vi "2019 deep space game Final.vi"() -> ()   [LabVIEW 2018]
panel:
  in  "Red Auto Points":dbl
  in  "Red End Game Points":dbl
  out "Red Score":dbl(slide) scale=0.0..200.0
  in  "Red Hatch":bool
  in  "Red Cargo":bool
  in  "Blue Foul":bool
  in  "Blue Tech Foul":bool
  out "Blue Score":dbl(slide) scale=0.0..200.0
  in  "Red Tech Foul":bool
  in  "Red Foul":bool
  in  "Blue End Game Points":dbl
  in  "Blue Auto Points":dbl
  in  "Blue Cargo":bool
  in  "Blue Hatch":bool
  out "Red Table of Pain":dbl[](array[numeric])
  out "Blue Table of Pain":dbl[](array[numeric])
  out "Thunder Down Under":T1
  out "SHARP":T1
  out "MARS":T1
  out "CIA":T1
  out "Cheezy Poofs":T1
  in  "End Game":bool
  out "Turn Number":i32(slide) scale=0.0..30.0
  in  "Next Turn":bool
  out "Krios":T1
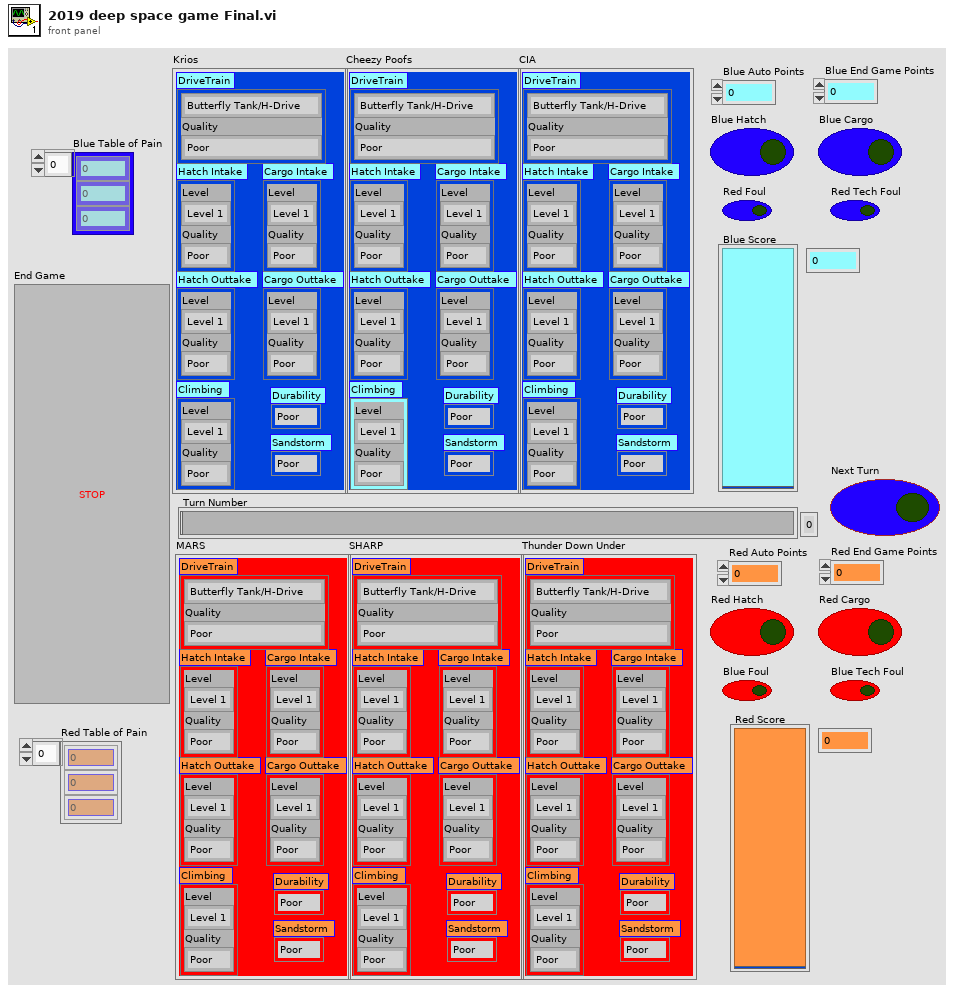
[diagram p1: front panel]
types:
  T1 = cluster{"DriveTrain":cluster{enum16{"Butterfly Tank/H-Drive", "Butterfly-Tank/Tank", "Tread", "Strafe", "Swerve", "Tank Traction"}, "Quality":enum16{"Poor", "Good", "Excellent"}}, "Cargo Intake":cluster{"Level":enum16{"Level 1", "Level 2", "Level 3"}, "Quality":enum16{"Poor", "Good", "Excellent"}}, "Hatch Intake":cluster{"Level":enum16{"Level 1", "Level 2", "Level 3"}, "Quality":enum16{"Poor", "Good", "Excellent"}}, "Cargo Outtake":cluster{"Level":enum16{"Level 1", "Level 2", "Level 3"}, "Quality":enum16{"Poor", "Good", "Excellent"}}, "Hatch Outtake":cluster{"Level":enum16{"Level 1", "Level 2", "Level 3"}, "Quality":enum16{"Poor", "Good", "Excellent"}}, "Climbing":cluster{"Level":enum16{"Level 1", "Level 2", "Level 3"}, "Quality":enum16{"Poor", "Good", "Excellent"}}, "Durability":enum16{"Poor", "Good", "Excellent"}, "Sandstorm":enum16{"Poor", "Good", "Excellent"}}
  T2 = cluster{cluster{enum16{"Butterfly Tank/H-Drive", "Butterfly-Tank/Tank", "Tread", "Strafe", "Swerve", "Tank Traction"}, "y":enum16{"Poor", "Good", "Excellent"}}, cluster{"Level":enum16{"Level 1", "Level 2", "Level 3"}, "y":enum16{"Poor", "Good", "Excellent"}}, cluster{"Level":enum16{"Level 1", "Level 2", "Level 3"}, "y":enum16{"Poor", "Good", "Excellent"}}, cluster{"Level":enum16{"Level 1", "Level 2", "Level 3"}, "y":enum16{"Poor", "Good", "Excellent"}}, cluster{"Level":enum16{"Level 1", "Level 2", "Level 3"}, "y":enum16{"Poor", "Good", "Excellent"}}, "Climbing":cluster{"Level":enum16{"Level 1", "Level 2", "Level 3"}, "Quality":enum16{"Poor", "Good", "Excellent"}}, "Durability":enum16{"Poor", "Good", "Excellent"}, "Sandstorm":enum16{"Poor", "Good", "Excellent"}}
  T3 = cluster{"Sandstorm":cluster{cluster{enum16{"Butterfly Tank/H-Drive", "Butterfly-Tank/Tank", "Tread", "Strafe", "Swerve", "Tank Traction"}, "y":enum16{"Poor", "Good", "Excellent"}}, cluster{"Level":enum16{"Level 1", "Level 2", "Level 3"}, "y":enum16{"Poor", "Good", "Excellent"}}, cluster{"Level":enum16{"Level 1", "Level 2", "Level 3"}, "y":enum16{"Poor", "Good", "Excellent"}}, cluster{"Level":enum16{"Level 1", "Level 2", "Level 3"}, "y":enum16{"Poor", "Good", "Excellent"}}, cluster{"Level":enum16{"Level 1", "Level 2", "Level 3"}, "y":enum16{"Poor", "Good", "Excellent"}}, "Climbing":cluster{"Level":enum16{"Level 1", "Level 2", "Level 3"}, "Quality":enum16{"Poor", "Good", "Excellent"}}, "Durability":enum16{"Poor", "Good", "Excellent"}, "Sandstorm":enum16{"Poor", "Good", "Excellent"}}, "Sandstorm":cluster{cluster{enum16{"Butterfly Tank/H-Drive", "Butterfly-Tank/Tank", "Tread", "Strafe", "Swerve", "Tank Traction"}, "y":enum16{"Poor", "Good", "Excellent"}}, cluster{"Level":enum16{"Level 1", "Level 2", "Level 3"}, "y":enum16{"Poor", "Good", "Excellent"}}, cluster{"Level":enum16{"Level 1", "Level 2", "Level 3"}, "y":enum16{"Poor", "Good", "Excellent"}}, cluster{"Level":enum16{"Level 1", "Level 2", "Level 3"}, "y":enum16{"Poor", "Good", "Excellent"}}, cluster{"Level":enum16{"Level 1", "Level 2", "Level 3"}, "y":enum16{"Poor", "Good", "Excellent"}}, "Climbing":cluster{"Level":enum16{"Level 1", "Level 2", "Level 3"}, "Quality":enum16{"Poor", "Good", "Excellent"}}, "Durability":enum16{"Poor", "Good", "Excellent"}, "Sandstorm":enum16{"Poor", "Good", "Excellent"}}, "Sandstorm":cluster{cluster{enum16{"Butterfly Tank/H-Drive", "Butterfly-Tank/Tank", "Tread", "Strafe", "Swerve", "Tank Traction"}, "y":enum16{"Poor", "Good", "Excellent"}}, cluster{"Level":enum16{"Level 1", "Level 2", "Level 3"}, "y":enum16{"Poor", "Good", "Excellent"}}, cluster{"Level":enum16{"Level 1", "Level 2", "Level 3"}, "y":enum16{"Poor", "Good", "Excellent"}}, cluster{"Level":enum16{"Level 1", "Level 2", "Level 3"}, "y":enum16{"Poor", "Good", "Excellent"}}, cluster{"Level":enum16{"Level 1", "Level 2", "Level 3"}, "y":enum16{"Poor", "Good", "Excellent"}}, "Climbing":cluster{"Level":enum16{"Level 1", "Level 2", "Level 3"}, "Quality":enum16{"Poor", "Good", "Excellent"}}, "Durability":enum16{"Poor", "Good", "Excellent"}, "Sandstorm":enum16{"Poor", "Good", "Excellent"}}, "Sandstorm":cluster{cluster{enum16{"Butterfly Tank/H-Drive", "Butterfly-Tank/Tank", "Tread", "Strafe", "Swerve", "Tank Traction"}, "y":enum16{"Poor", "Good", "Excellent"}}, cluster{"Level":enum16{"Level 1", "Level 2", "Level 3"}, "y":enum16{"Poor", "Good", "Excellent"}}, cluster{"Level":enum16{"Level 1", "Level 2", "Level 3"}, "y":enum16{"Poor", "Good", "Excellent"}}, cluster{"Level":enum16{"Level 1", "Level 2", "Level 3"}, "y":enum16{"Poor", "Good", "Excellent"}}, cluster{"Level":enum16{"Level 1", "Level 2", "Level 3"}, "y":enum16{"Poor", "Good", "Excellent"}}, "Climbing":cluster{"Level":enum16{"Level 1", "Level 2", "Level 3"}, "Quality":enum16{"Poor", "Good", "Excellent"}}, "Durability":enum16{"Poor", "Good", "Excellent"}, "Sandstorm":enum16{"Poor", "Good", "Excellent"}}, "Sandstorm":cluster{cluster{enum16{"Butterfly Tank/H-Drive", "Butterfly-Tank/Tank", "Tread", "Strafe", "Swerve", "Tank Traction"}, "y":enum16{"Poor", "Good", "Excellent"}}, cluster{"Level":enum16{"Level 1", "Level 2", "Level 3"}, "y":enum16{"Poor", "Good", "Excellent"}}, cluster{"Level":enum16{"Level 1", "Level 2", "Level 3"}, "y":enum16{"Poor", "Good", "Excellent"}}, cluster{"Level":enum16{"Level 1", "Level 2", "Level 3"}, "y":enum16{"Poor", "Good", "Excellent"}}, cluster{"Level":enum16{"Level 1", "Level 2", "Level 3"}, "y":enum16{"Poor", "Good", "Excellent"}}, "Climbing":cluster{"Level":enum16{"Level 1", "Level 2", "Level 3"}, "Quality":enum16{"Poor", "Good", "Excellent"}}, "Durability":enum16{"Poor", "Good", "Excellent"}, "Sandstorm":enum16{"Poor", "Good", "Excellent"}}, "Sandstorm":cluster{cluster{enum16{"Butterfly Tank/H-Drive", "Butterfly-Tank/Tank", "Tread", "Strafe", "Swerve", "Tank Traction"}, "y":enum16{"Poor", "Good", "Excellent"}}, cluster{"Level":enum16{"Level 1", "Level 2", "Level 3"}, "y":enum16{"Poor", "Good", "Excellent"}}, cluster{"Level":enum16{"Level 1", "Level 2", "Level 3"}, "y":enum16{"Poor", "Good", "Excellent"}}, cluster{"Level":enum16{"Level 1", "Level 2", "Level 3"}, "y":enum16{"Poor", "Good", "Excellent"}}, cluster{"Level":enum16{"Level 1", "Level 2", "Level 3"}, "y":enum16{"Poor", "Good", "Excellent"}}, "Climbing":cluster{"Level":enum16{"Level 1", "Level 2", "Level 3"}, "Quality":enum16{"Poor", "Good", "Excellent"}}, "Durability":enum16{"Poor", "Good", "Excellent"}, "Sandstorm":enum16{"Poor", "Good", "Excellent"}}}
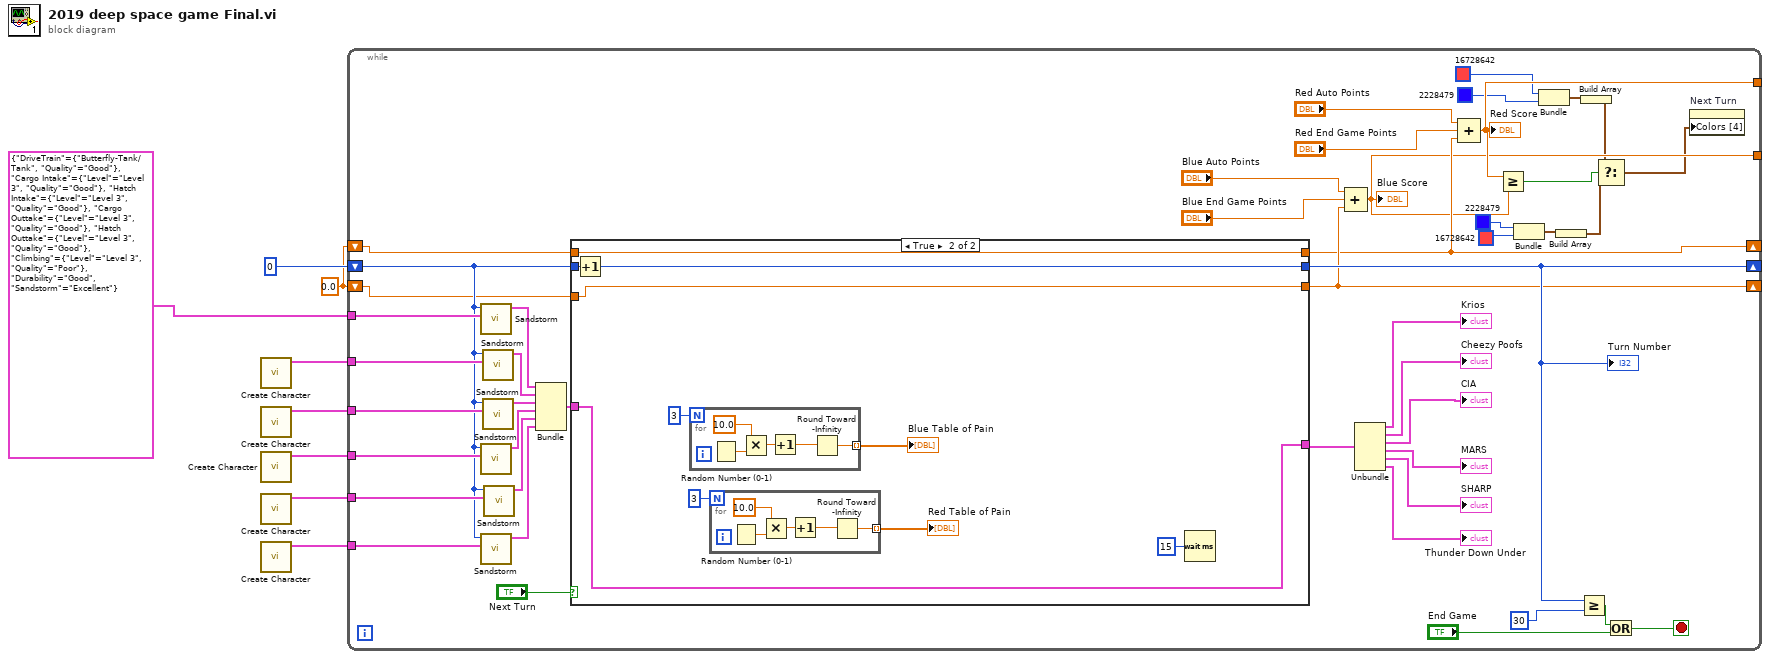
[diagram p0: block diagram]
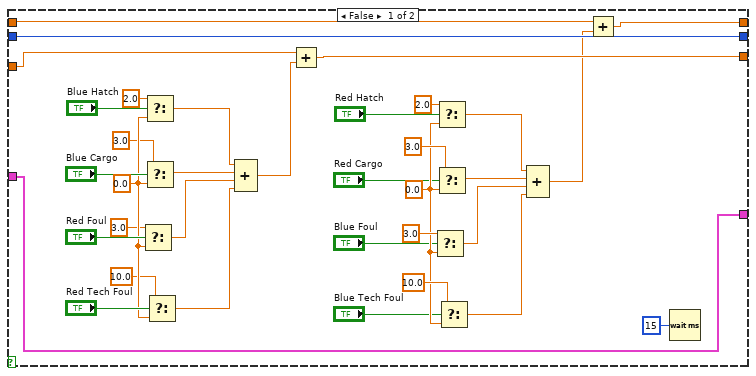
[diagram p2: hidden frame]
diagram:
  w2 = 0.0
  n1 = call "Create Character.vi"() -> ("Normal Game"=w7:T1)  [unwired: 11 in]
  n2 = call "Create Character.vi"() -> ("Normal Game"=w6:T1)  [unwired: 11 in]
  n3 = call "Create Character.vi"() -> ("Normal Game"=w5:T1)  [unwired: 11 in]
  n4 = call "Create Character.vi"() -> ("Normal Game"=w4:T1)  [unwired: 11 in]
  n5 = call "Create Character.vi"() -> ("Normal Game"=w3:T1)  [unwired: 11 in]
  n6 = while {
    shift-right: [w50] -> _
    shift-left: 0 -> [w43]
    tunnel: T1 {"DriveTrain"={enum."Butterfly-Tank/Tank", "Quality"=enum."Good"}, "Cargo Intake"={"Level"=enum."Level 3", "Quality"=enum."Good"}, "Hatch Intake"={"Level"=enum."Level 3", "Quality"=enum."Good"}, "Cargo Outtake"={"Level"=enum."Level 3", "Quality"=enum."Good"}, "Hatch Outtake"={"Level"=enum."Level 3", "Quality"=enum."Good"}, "Climbing"={"Level"=enum."Level 3", "Quality"=enum."Poor"}, "Durability"=enum."Good", "Sandstorm"=enum."Excellent"} ("Normal Game") -> [w44]
    tunnel: w7 -> [w45]
    tunnel: w6 -> [w46]
    tunnel: w5 -> [w47]
    tunnel: w4 -> [w48]
    tunnel: w3 -> [w49]
    shift-right: [w21] -> _
    shift-left: w2 -> [w28]
    shift-right: [w26] -> _
    shift-left: w2 -> [w27]
    tunnel: [w19] -> _
    tunnel: [w18] -> _
    stop <- w54 stop-if-true
    n7 = call "Sandstorm.vi"("Normal Game"=w44, "Turn Number in"=w43) -> ("Sandstorm"=w42:T2)  [unwired: 9 in]
    n8 = call "Sandstorm.vi"("Normal Game"=w47, "Turn Number in"=w43) -> ("Sandstorm"=w37:T2)  [unwired: 9 in]
    n9 = call "Sandstorm.vi"("Normal Game"=w49, "Turn Number in"=w43) -> ("Sandstorm"=w39:T2)  [unwired: 9 in]
    n10 = call "Sandstorm.vi"("Normal Game"=w45, "Turn Number in"=w43) -> ("Sandstorm"=w41:T2)  [unwired: 9 in]
    n11 = call "Sandstorm.vi"("Normal Game"=w46, "Turn Number in"=w43) -> ("Sandstorm"=w40:T2)  [unwired: 9 in]
    n12 = call "Sandstorm.vi"("Normal Game"=w48, "Turn Number in"=w43) -> ("Sandstorm"=w38:T2)  [unwired: 9 in]
    n13 = Bundle("Sandstorm"=w42, "Sandstorm"=w41, "Sandstorm"=w40, "Sandstorm"=w37, "Sandstorm"=w38, "Sandstorm"=w39) -> (w36:T3)  [unwired: 1 in]
    n14 = case shown="True" "Next Turn" {
      tunnel: w43 -> [w90 w100]
      tunnel: [w90 w99] -> w50
      tunnel: w36 -> [w88 w97]
      tunnel: [w88 w97] -> w35
      tunnel: w28 -> [w57 w92]
      tunnel: w27 -> [w74 w91]
      tunnel: [w56 w92] -> w21
      tunnel: [w72 w91] -> w26
      frame False {
        w62 = 0.0 ("f")
        w83 = 0.0 ("f")
        n15 = Select(t=3.0, s="Red Foul", f=w83) -> (s? t:f=w76:dbl)
        n16 = Select(t=2.0, s="Blue Hatch", f=w83) -> (s? t:f=w78:dbl)
        n17 = Select(t=3.0, s="Blue Cargo", f=w83) -> (s? t:f=w77:dbl)
        n18 = Select(t=10.0, s="Red Tech Foul", f=w83) -> (s? t:f=w75:dbl)
        n19 = Compound Arithmetic op=ADD(w78, w77, w76, w75) -> (w73:dbl)
        n20 = Add(x=w74, y=w73) -> (x+y=w72:dbl)
        n21 = Select(t=3.0, s="Blue Foul", f=w62) -> (s? t:f=w69:dbl)
        n22 = Select(t=2.0, s="Red Hatch", f=w62) -> (s? t:f=w67:dbl)
        n23 = Select(t=3.0, s="Red Cargo", f=w62) -> (s? t:f=w68:dbl)
        n24 = Select(t=10.0, s="Blue Tech Foul", f=w62) -> (s? t:f=w70:dbl)
        n25 = Compound Arithmetic op=ADD(w67, w68, w69, w70) -> (w71:dbl)
        n26 = Add(x=w57, y=w71) -> (x+y=w56:dbl)
        n27 = Wait (ms)(milliseconds to wait=u32 15) -> ()  [unwired: 1 out]
      }
      frame True {
        n28 = Increment(x=w100) -> (x+1=w99:i32)
        n29 = for {
          N: 3 -> [_]
          tunnel: [w108] -> w95 mode=indexing
          n30 = Random Number (0-1)() -> (number: 0 to 1=w110:dbl)
          n31 = Multiply(x=10.0, y=w110) -> (x*y=w107:dbl)
          n32 = Increment(x=w107) -> (x+1=w106:dbl)
          n33 = Round Toward -Infinity(1:w106) -> (0:w108:dbl)
        }
        "Blue Table of Pain" <- w95
        n34 = for {
          N: 3 -> [_]
          tunnel: [w103] -> w94 mode=indexing
          n35 = Random Number (0-1)() -> (number: 0 to 1=w105:dbl)
          n36 = Multiply(x=10.0, y=w105) -> (x*y=w102:dbl)
          n37 = Increment(x=w102) -> (x+1=w101:dbl)
          n38 = Round Toward -Infinity(1:w101) -> (0:w103:dbl)
        }
        "Red Table of Pain" <- w94
        n39 = Wait (ms)(milliseconds to wait=u32 15) -> ()  [unwired: 1 out]
      }
    }
    "Turn Number" <- w50
    n40 = Compound Arithmetic op=ADD("Blue Auto Points", "Blue End Game Points", w26) -> (w18:dbl)
    "Blue Score" <- w18
    n41 = Unbundle(w35) -> ("Sandstorm"=→"Krios":T2, "Sandstorm"=→"Cheezy Poofs":T2, "Sandstorm"=→"CIA":T2, "Sandstorm"=→"MARS":T2, "Sandstorm"=→"SHARP":T2, "Sandstorm"=→"Thunder Down Under":T2)
    n42 = Compound Arithmetic op=ADD("Red Auto Points", "Red End Game Points", w21) -> (w19:dbl)
    "Red Score" <- w19
    n43 = Greater Or Equal?(x=w19, y=w18) -> (x >= y?=w14:bool)
    n44 = Bundle(u32 2228479, u32 16728642) -> (w13:cluster{u32, u32})  [unwired: 1 in]
    n45 = Bundle(u32 16728642, u32 2228479) -> (w20:cluster{u32, u32})  [unwired: 1 in]
    n46 = Build Array(w13) -> (w10:cluster{u32, u32}[])
    n47 = Greater Or Equal?(x=w50, y=30) -> (x >= y?=w53:bool)
    n48 = Build Array(w20) -> (w15:cluster{u32, u32}[])
    n49 = Select(t=w15, s=w14, f=w10) -> (s? t:f=w9:cluster{u32, u32}[])
    n50 = Or(x=w53, y="End Game") -> (x .or. y?=w54:bool)
    n51 = property on="Next Turn" class="Bool"("Colors [4]"=w9) -> ()  [unwired: 2 in, 2 out]
  }
